vi "select_wavelength.vi"(0 "wavelength":dbl, 1 "Spectrometer Handle in 2":i16=1 min=1 max=100 step=1, 3 "monochromator error in":errorcluster) -> (8 "Spectrometer Handle out":i16=1 min=1 max=100 step=1, 10 "monochromator error out":errorcluster)   [LabVIEW 2016]
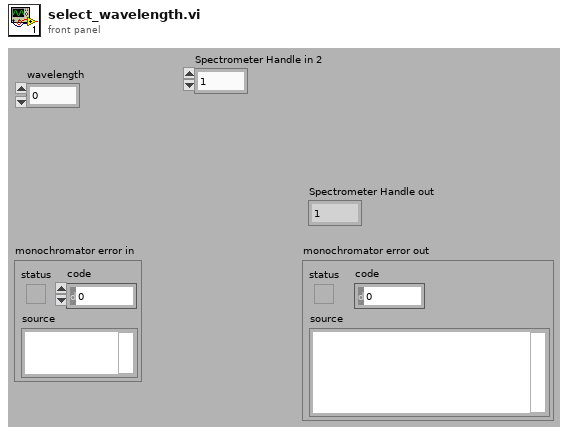
[diagram p1: front panel]
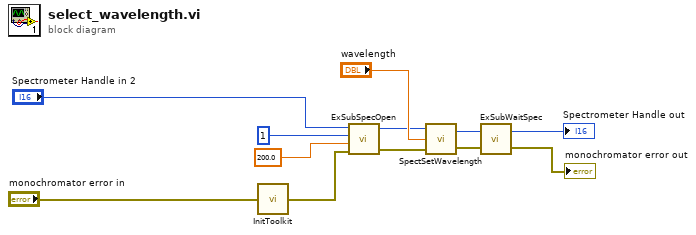
[diagram p0: block diagram]
diagram:
  n1 = call <userlib>:"InitToolkit.vi"("error in"="monochromator error in") -> ("error out"=w6:errorcluster)
  n2 = call "ExSubSpecOpen.vi"("error in (no error)"=w6, "Grating speed"=200.0, "Grating number"=1, "Camera Handles"="Spectrometer Handle in 2") -> ("error out"=w1:errorcluster, "Spectrometer Handle"=w4:u32)  [unwired: 1 out]
  n3 = call <userlib>:"SpectSetWavelength.vi"("error in"=w1, "Wavelength"="wavelength", "Spectrometer Handle"=w4) -> ("error out"=w11:errorcluster, "Spectrumeter Handle"=w12:u32)
  n4 = call "ExSubWaitSpec.vi"("error in (no error)"=w11, "Spectrometer Handle"=w12) -> ("error out"=→"monochromator error out":errorcluster, "Spectrometer handle"=→"Spectrometer Handle out":u32)
